vi "Add Comp Prompt.vi"() -> (2 "Cancelled":bool, 3 "Selected Component":refnum<class "Item.lvclass">)   [LabVIEW 2020, in "App.lvclass"]
uses:
  App.lvclass
  Item/Item.lvclass
  Battery Stack/Battery Stack.lvclass
  C:/dev/IlluminatedG/lv-oopanel-gc-calc/Item/Item.lvclass
  LED Array/LED Array.lvclass
  LED Matrix/LED Matrix.lvclass
  Logic Circuit/Logic Circuit.lvclass
  Metal Case/Metal Case.lvclass
  Simple Case/Simple Case.lvclass
  Simple Circuit/Simple Circuit.lvclass
  Single Cell Battery/Single Cell Battery.lvclass
  Small Register Bank/Small Register Bank.lvclass
  Wooden Case/Wooden Case.lvclass
panel:
  in  "Cancel":bool
  in  "OK":bool
  in  "Component":string(combo)
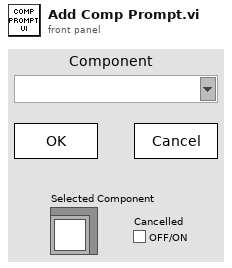
[diagram p1: front panel]
types:
  T1 = cluster{"class name":string, "LED Array.lvclass":refnum<class "Item.lvclass">}
  T2 = cluster{"class name":string, "LED Array.lvclass":refnum<class "Item.lvclass">}[]
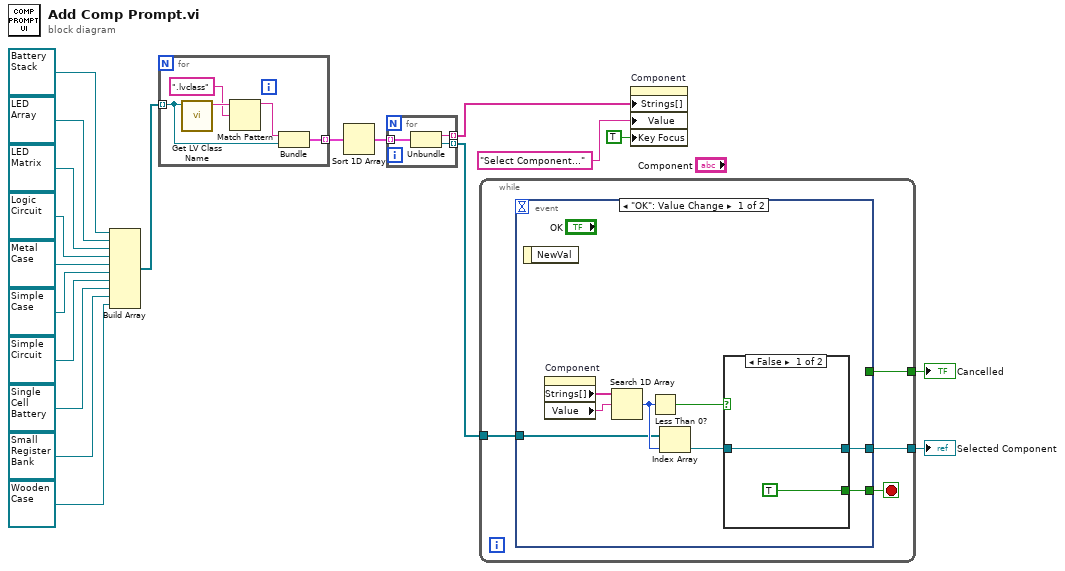
[diagram p0: block diagram]
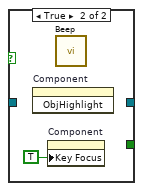
[diagram p2: hidden frame]
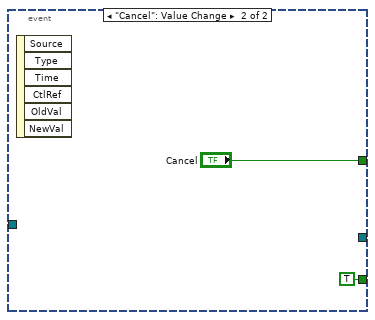
[diagram p3: hidden frame]
diagram:
  n1 = Build Array(refnum<class "Battery Stack.lvclass"> refnum ("Battery Stack.lvclass"), refnum<class "LED Array.lvclass"> refnum ("LED Array.lvclass"), refnum<class "LED Matrix.lvclass"> refnum ("LED Matrix.lvclass"), refnum<class "Logic Circuit.lvclass"> refnum ("Logic Circuit.lvclass"), refnum<class "Metal Case.lvclass"> refnum ("Metal Case.lvclass"), refnum<class "Simple Case.lvclass"> refnum ("Simple Case.lvclass"), refnum<class "Simple Circuit.lvclass"> refnum ("Simple Circuit.lvclass"), refnum<class "Single Cell Battery.lvclass"> refnum ("Single Cell Battery.lvclass"), refnum<class "Small Register Bank.lvclass"> refnum ("Small Register Bank.lvclass"), refnum<class "Wooden Case.lvclass"> refnum ("Wooden Case.lvclass")) -> (w8:refnum<class "Item.lvclass">[])
  n2 = for {
    tunnel: w8 -> [w21] mode=indexing
    tunnel: [w20] -> w6 mode=indexing
    n3 = call <vilib>:"Get LV Class Name.vi"("object"=w21) -> ("class name"=w24:string)  [unwired: 9 in, 1 out]
    n4 = Match Pattern(string=w24, regular expression=".lvclass") -> (before substring=w22:string)  [unwired: 1 in, 3 out]
    n5 = Bundle("class name"=w22, "LED Array.lvclass"=w21) -> (w20:T1)  [unwired: 1 in]
  }
  n6 = Sort 1D Array(array=w6) -> (sorted array=w5:T2)
  n7 = for {
    tunnel: w5 -> [w27] mode=indexing
    tunnel: [w26] -> w3 mode=indexing
    tunnel: [w25] -> w4 mode=indexing
    n8 = Unbundle(w27) -> ("class name"=w25:string, "LED Array.lvclass"=w26:refnum<class "Item.lvclass">)
  }
  n9 = while {
    tunnel: w3 -> [w30]
    tunnel: [w29] -> w2
    tunnel: [w28] -> w1
    stop <- w31 stop-if-true
    n10 = event shown="[0] \"OK\": Value Change" {
      selector: _ -> [_ _]
      dyn-events: _ -> [_ _]
      timeout: _ -> [_ _]
      tunnel: [w35 TRUE] -> w31
      tunnel: w30 -> [w34 _]
      tunnel: [_ "Cancel"] -> w29
      tunnel: [w32 _] -> w28
      event "OK": Value Change {
        n11 = event-data() -> ()  [unwired: 1 in, 1 out]
        n12 = property on="Component" class="CmbBox"() -> ("Strings[]"=w39:string[], "Value"=w38:string)  [unwired: 2 in, 2 out]
        n13 = Search 1D Array(1D array=w39, element=w38) -> (index of element=w37:i32)  [unwired: 1 in]
        n14 = Less Than 0?(x=w37) -> (x < 0?=w36:bool)
        n15 = Index Array(array=w34, index=w37) -> (element=w33:refnum<class "Item.lvclass">)
        n16 = case shown="False" w36 {
          tunnel: [TRUE _] -> w35
          tunnel: w33 -> [w40 _]
          tunnel: [w40 _] -> w32
          frame False {
          }
          frame True {
            n17 = invoke on="Component" class="CmbBox" method="ObjHighlight"() -> ()  [unwired: 3 in, 3 out]
            n18 = property on="Component" class="CmbBox"("Key Focus"=TRUE) -> ()  [unwired: 2 in, 2 out]
            n19 = call <vilib>:"Beep.vi"() -> ()  [unwired: 12 in]
          }
        }
      }
      event "Cancel": Value Change {
        n20 = event-data() -> ()  [unwired: 1 in, 6 out]
      }
    }
  }
  "Cancelled" <- w2
  "Selected Component" <- w1
  n21 = property on="Component" class="CmbBox"("Strings[]"=w4, "Value"="Select Component...", "Key Focus"=TRUE) -> ()  [unwired: 2 in, 2 out]
